vi "Agilent Channels.vi"(0 "file path (dialog if empty)":path=path "C:/NI-2010/Trunk/Dryer Wilt/Agilent Channel Assignment - Wilt.ini") -> (3 "Temperature Channels":T1[](array[typedef]), 4 "Station Data Headers":string[][](array[string]), 6 "Index Array":i32[][](array[numeric]), 8 "Agilent Channels Raw":T1[](array[typedef]), 10 "Agilent Channels To Read":T1[](array[typedef]), 14 "Start Buttons":T1[](array[typedef]), 15 "Agilent Channel Water Valves":T1[](array[typedef]))   [LabVIEW 2012]
uses:
  Agilent Channel Definition.ctl
  <vilib>/Utility/file.llb/Read From Spreadsheet File (string).vi
panel:
  out "Array":i32[](array[numeric])
  out "Agilent6 Channels":string[][](array[string])
  out "Agilent5 Channels":string[][](array[string])
  out "Agilent4 Channels":string[][](array[string])
  out "Agilent3 Channels":string[][](array[string])
  out "Agilent2 Channels":string[][](array[string])
  out "Agilent1 Channels":string[][](array[string])
  out "all rows":string[][](array[string])
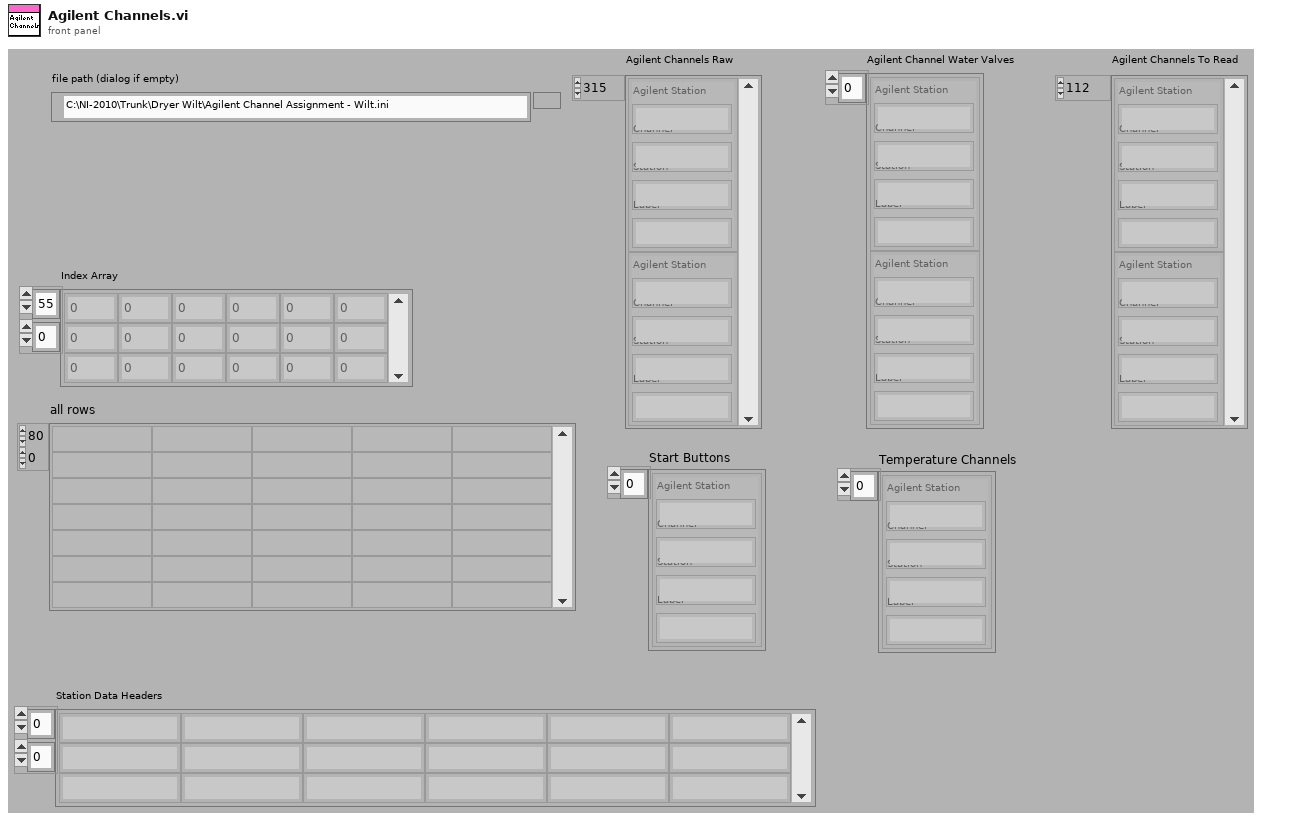
[diagram p1: front panel]
types:
  T1 = typedef "Agilent Channel Definition.ctl" = cluster{"Channel":string, "Station":string, "Label":string, "Agilent Station":string}
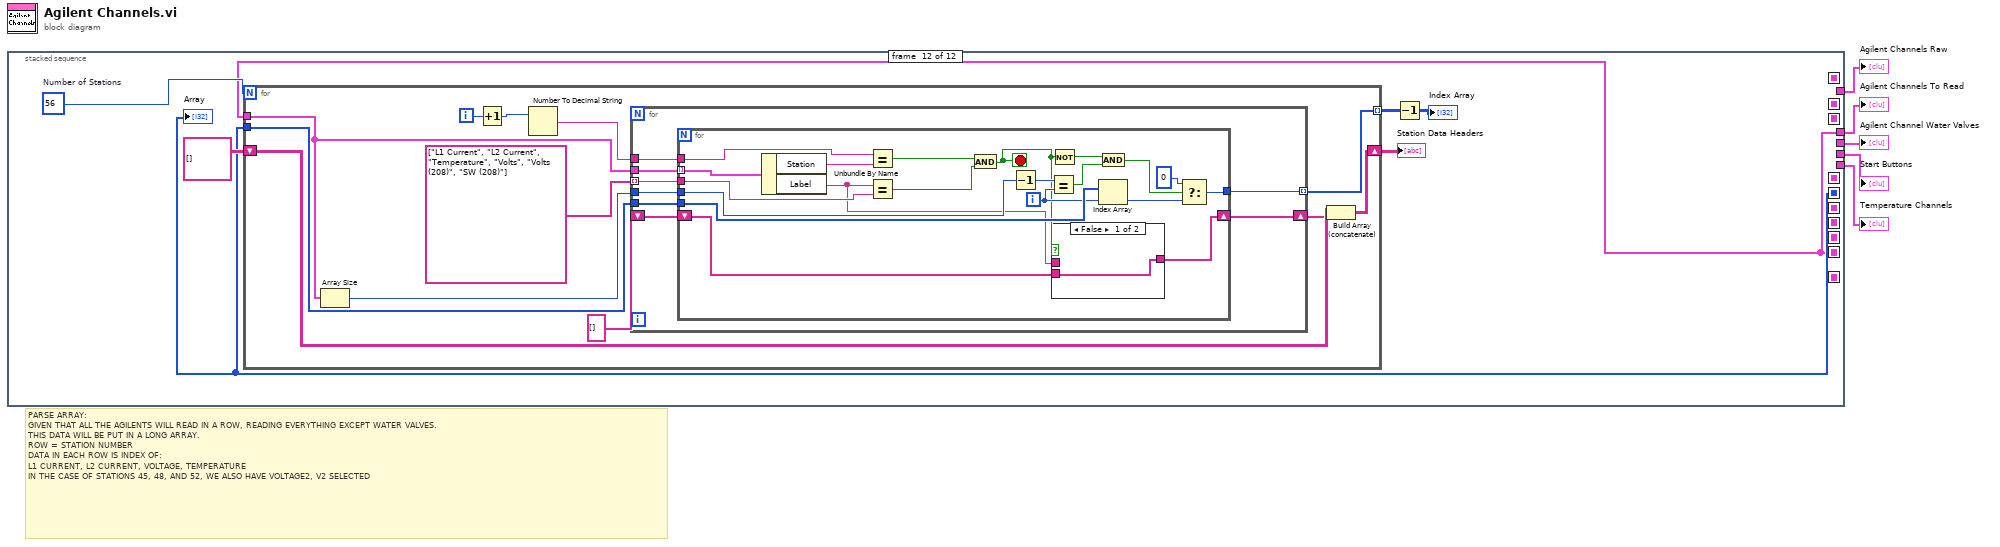
[diagram p0: block diagram]
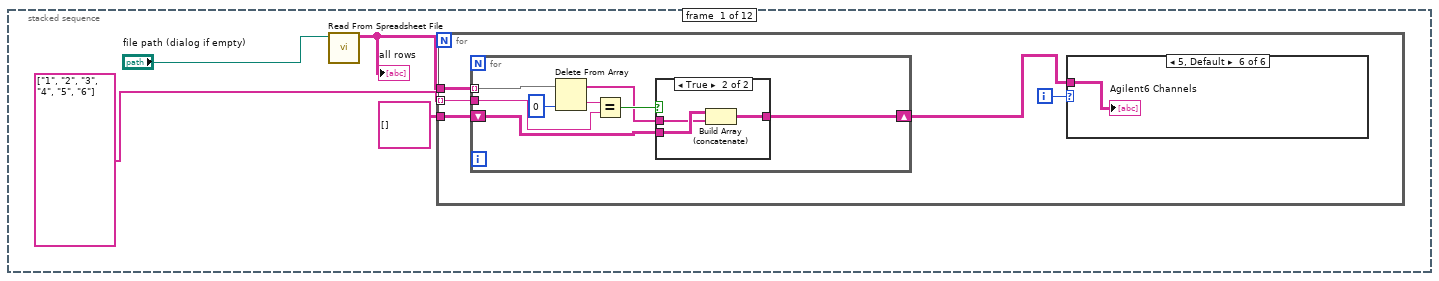
[diagram p2: hidden frame]
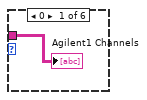
[diagram p3: hidden frame]
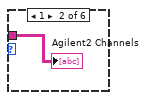
[diagram p4: hidden frame]
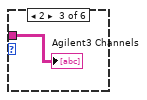
[diagram p5: hidden frame]
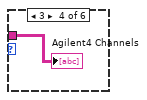
[diagram p6: hidden frame]
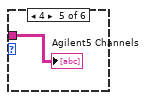
[diagram p7: hidden frame]
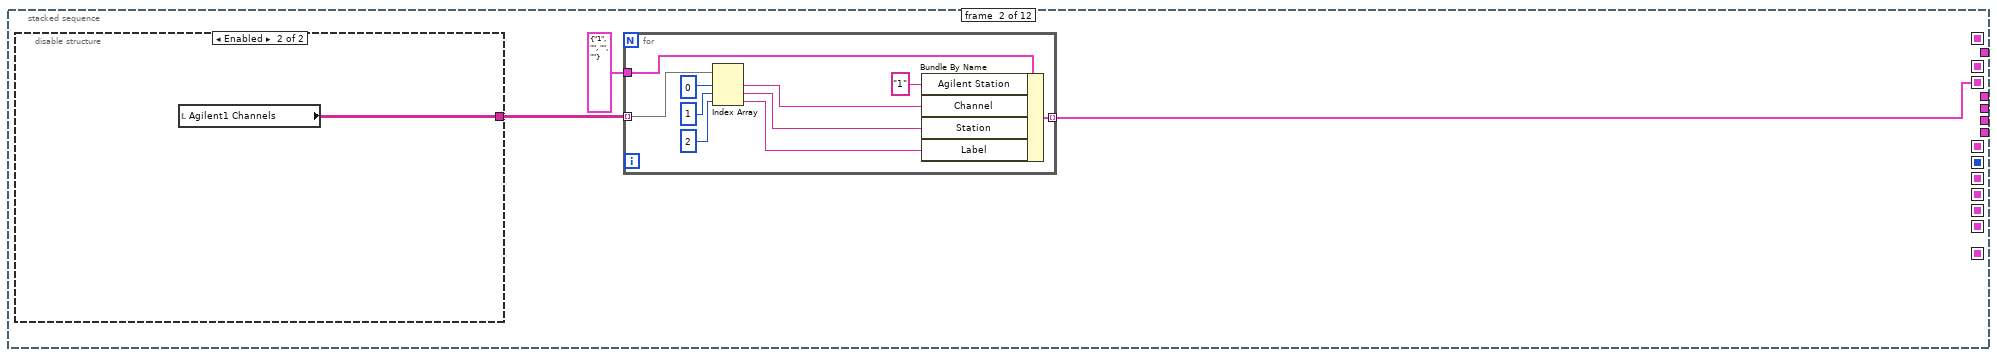
[diagram p9: hidden frame]
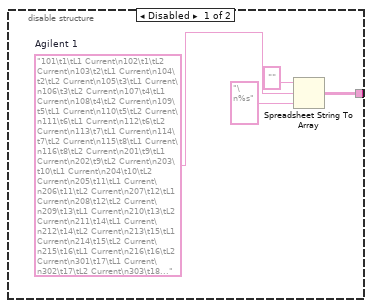
[diagram p10: hidden frame]
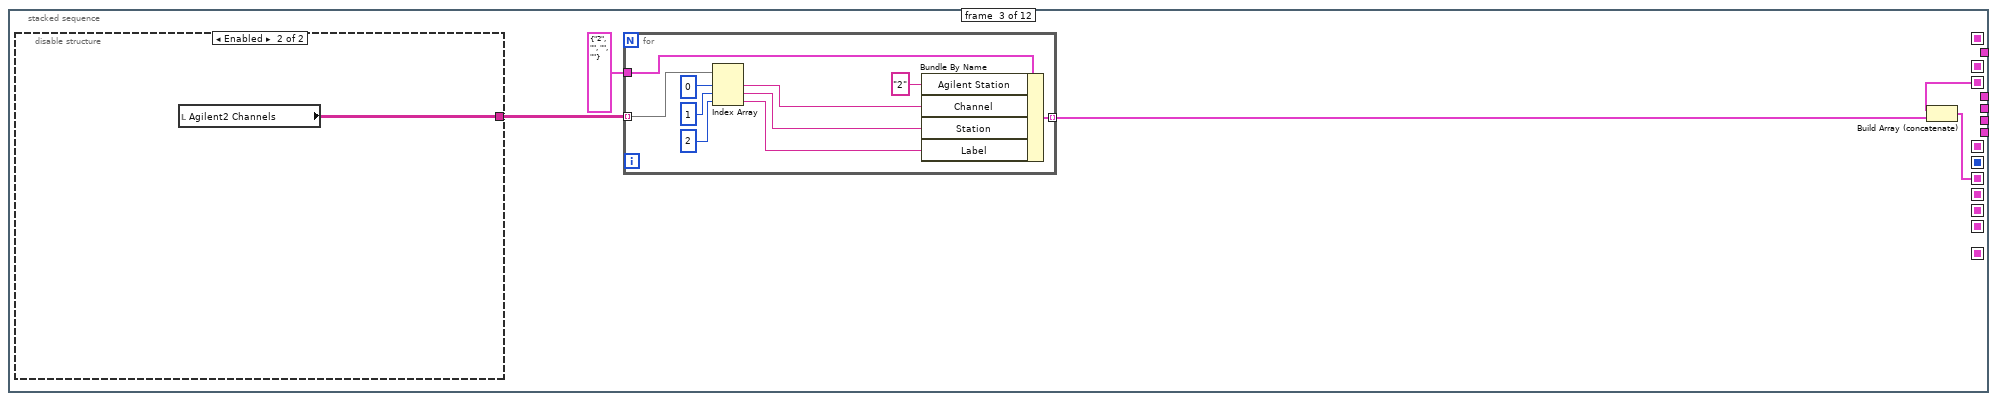
[diagram p11: hidden frame]
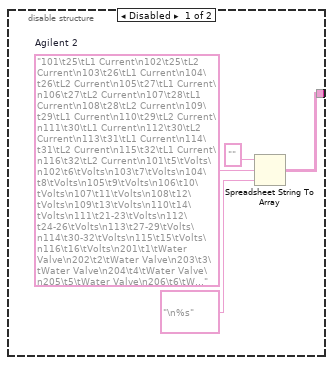
[diagram p12: hidden frame]
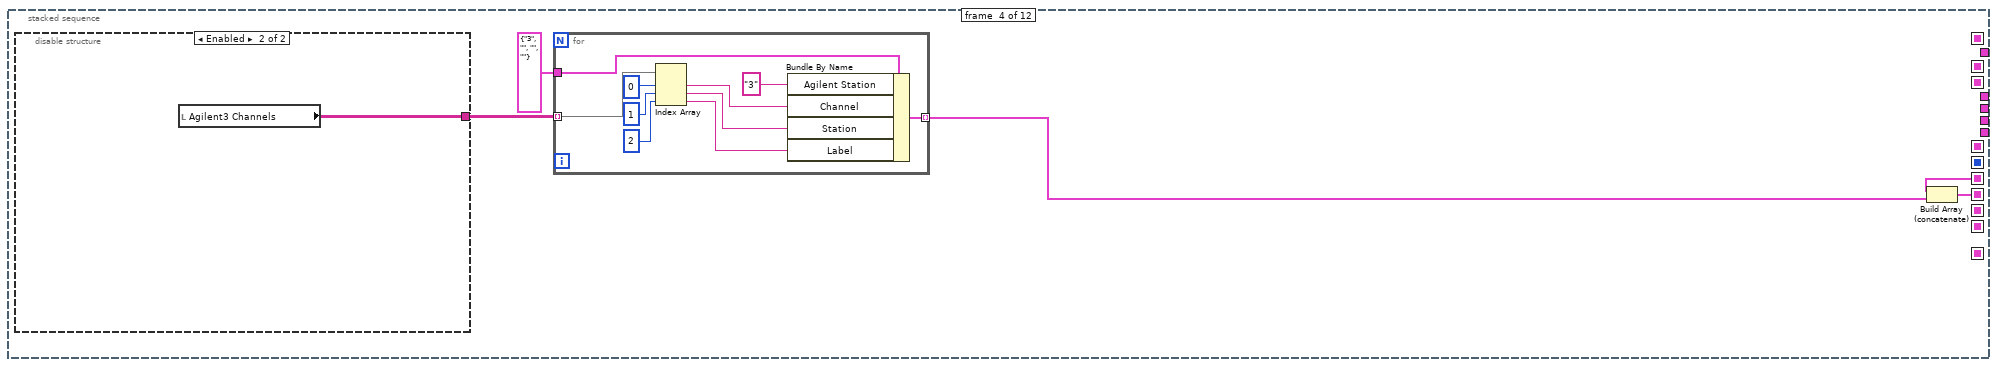
[diagram p13: hidden frame]
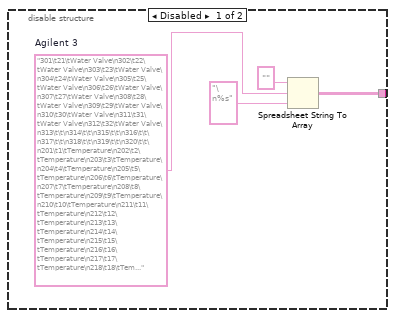
[diagram p14: hidden frame]
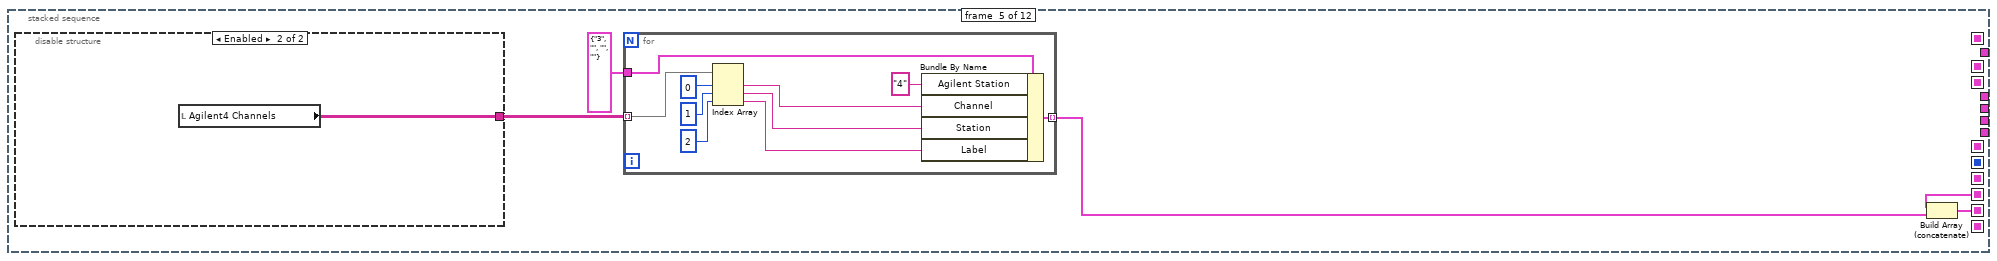
[diagram p15: hidden frame]
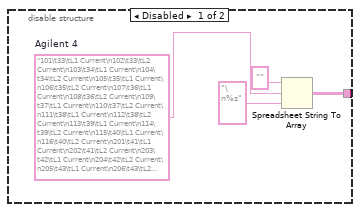
[diagram p16: hidden frame]
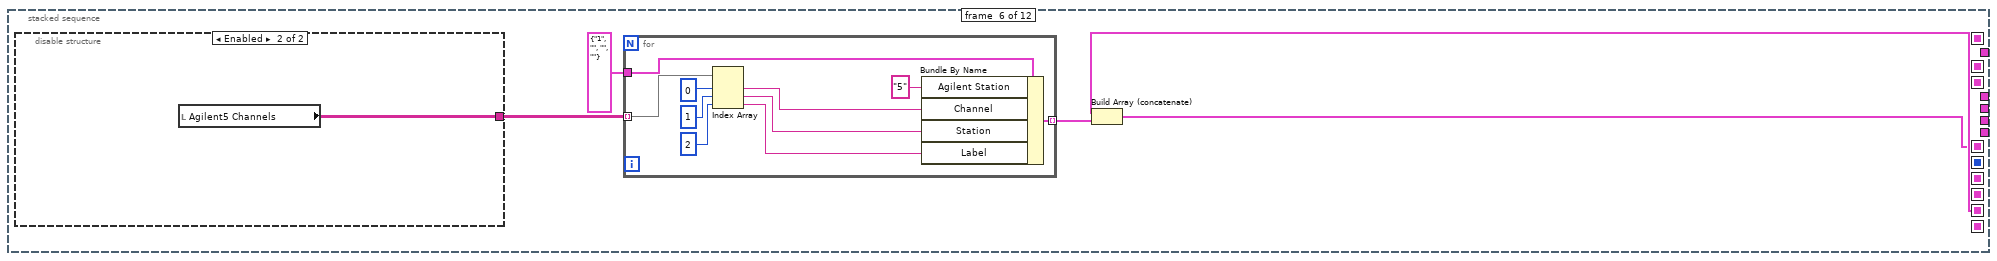
[diagram p17: hidden frame]
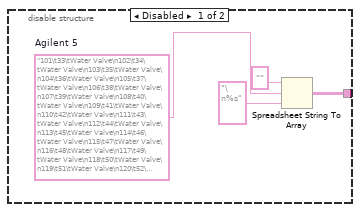
[diagram p18: hidden frame]
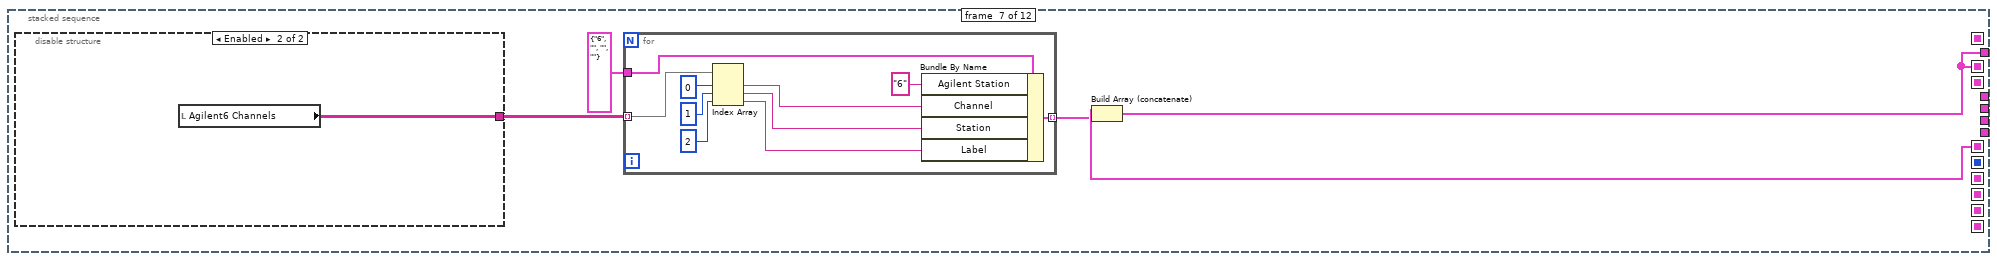
[diagram p19: hidden frame]
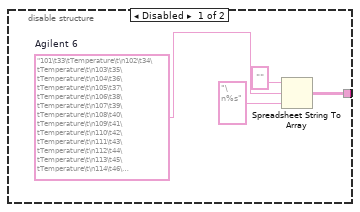
[diagram p20: hidden frame]
diagram:
  # "PARSE ARRAY:\nGIVEN THAT ALL THE AGILENTS WILL READ IN A ROW, READING EVERYTHING EXCEPT WATER VALVES.\nTHIS DATA WILL BE PUT IN A LONG ARRAY.\nROW = STATION NUMBER\nDATA IN EACH ROW IS INDEX OF:\nL1 CURRENT, L2 CURRENT, VOLTAGE, TEMPERATURE\nIN THE CASE OF STATIONS 45, 48, AND 52, WE ALSO HAVE VOLTAGE2, V2 SELECTED"
  n1 = stacked-sequence {
    seq-local: [_ w33 _ _ _ _ _ _ _ _ _ _] -> [_ _ w55 _ _ _ _ _ _ _ _ _]
    seq-local: [_ _ w54 _ _ _ _ _ _ _ _ _] -> [_ _ _ w75 _ _ _ _ _ _ _ _]
    seq-local: [_ _ _ w74 _ _ _ _ _ _ _ _] -> [_ _ _ _ w95 _ _ _ _ _ _ _]
    seq-local: [_ _ _ _ w94 _ _ _ _ _ _ _] -> [_ _ _ _ _ w115 _ _ _ _ _ _]
    seq-local: [_ _ _ _ _ w114 _ _ _ _ _ _] -> [_ _ _ _ _ _ w135 _ _ _ _ _]
    seq-local: [_ _ _ _ _ _ _ w154 _ _ _ _] -> [_ _ _ _ _ _ _ _ w173 _ _ _]
    seq-local: [_ _ _ _ _ _ _ _ _ _ w208 _] -> [_ _ _ _ _ _ _ _ _ _ _ w258]
    seq-local: [_ _ _ _ _ _ w131 _ _ _ _ _] -> [_ _ _ _ _ _ _ w153 _ w193 _ _]
    seq-local: [_ _ _ _ _ _ _ _ _ _ w206 _] -> [_ _ _ _ _ _ _ _ _ _ _ w261]
    seq-local: [_ _ _ _ _ _ _ _ w171 _ _ _] -> [_ _ _ _ _ _ _ _ _ _ w204 _]
    tunnel: [_ _ _ _ _ _ w131 _ _ _ _ _] -> w5
    tunnel: [_ _ _ _ _ _ _ _ _ _ _ w258] -> w4
    tunnel: [_ _ _ _ _ _ _ w151 _ _ _ _] -> w3
    tunnel: [_ _ _ _ _ _ _ _ w174 _ _ _] -> w2
    tunnel: [_ _ _ _ _ _ _ _ _ w191 _ _] -> w1
    frame #0 {
      n2 = call-poly <vilib>:"Read From Spreadsheet File.vi"("file path (dialog if empty)"="file path (dialog if empty)") -> ("all rows"=w8:string[][])  [unwired: 6 in, 4 out]
      "all rows" <- w8
      n3 = for {
        tunnel: w8 -> [w14]
        tunnel: string[][] [] -> [w12]
        tunnel: string[] ["1", "2", "3", "4", "5", "6"] -> [w11] mode=indexing
        i -> [w10]
        n4 = for {
          tunnel: w14 -> [w28] mode=indexing
          shift-right: [w24] -> w13
          shift-left: w12 -> [w23]
          tunnel: w11 -> [w21]
          n5 = Delete From Array(array=w28, index=0) -> (deleted portion=w26:string, array with subset deleted=w22:string[])  [unwired: 1 in]
          n6 = Equal?(x=w26, y=w21) -> (x = y?=w25:bool)
          n7 = case shown="True" w25 {
            tunnel: [w29 w32] -> w24
            tunnel: w23 -> [w29 w31]
            tunnel: w22 -> [_ w30]
            frame False {
            }
            frame True {
              n8 = Build Array (concatenate)(w31, w30) -> (w32:string[][])
            }
          }
        }
        n9 = case shown="5, Default" w10 {
          tunnel: w13 -> [w15 w16 w17 w18 w19 w20]
          frame 0 {
            "Agilent1 Channels" <- w15
          }
          frame 1 {
            "Agilent2 Channels" <- w16
          }
          frame 2 {
            "Agilent3 Channels" <- w17
          }
          frame 3 {
            "Agilent4 Channels" <- w18
          }
          frame 4 {
            "Agilent5 Channels" <- w19
          }
          frame 5, Default {
            "Agilent6 Channels" <- w20
          }
        }
      }
    }
    frame #1 {
      n10 = disable-structure shown="Enabled" {
        disable-tunnel: [w38 w40] -> w35
        frame Disabled {
          w36 = "101\t1\tL1 Current\n102\t1\tL2 Current\n103\t2\tL1 Current\n104\t2\tL2 Current\n105\t3\tL1 Current\n106\t3\tL2 Current\n107\t4\tL1 Current\n108\t4\tL2 Current\n109\t5\tL1 Current\n110\t5\tL2 Current\n111\t6\tL1 Current\n112\t6\tL2 Current\n113\t7\tL1 Current\n114\t7\tL2 Current\n115\t8\tL1 Current\n116\t8\tL2 Current\n201\t9\tL1 Current\n202\t9\tL2 Current\n203\t10\tL1 Current\n204\t10\tL2 Current\n205\t11\tL1 Current\n206\t11\tL2 Current\n207\t12\tL1 Current\n208\t12\tL2 Current\n209\t13\tL1 Current\n210\t13\tL2 Current\n211\t14\tL1 Current\n212\t14\tL2 Current\n213\t15\tL1 Current\n214\t15\tL2 Current\n215\t16\tL1 Current\n216\t16\tL2 Current\n301\t17\tL1 Current\n302\t17\tL2 Current\n303\t18\tL1 Current\n304\t18\tL2 Current\n305\t19\tL1 Current\n306\t19\tL2 Current\n307\t20\tL1 Current\n308\t20\tL2 Current\n309\t21\tL1 Current\n310\t21\tL2 Current\n311\t22\tL1 Current\n312\t22\tL2 Current\n313\t23\tL1 Current\n314\t23\tL2 Current\n315\t24\tL1 Current\n316\t24\tL2 Current"  # Agilent 1
          n11 = Spreadsheet String To Array(format string="", spreadsheet string=w36, array type (2D Dbl)="\n%s" ("format string")) -> (array=w38:string[][])  [unwired: 1 in]
        }
        frame Enabled {
          n12 = local read "Agilent1 Channels"() -> (w40:string[][])
        }
      }
      n13 = for {
        tunnel: w35 -> [w48] mode=indexing
        tunnel: T1 {"Channel"="1", "Station"="", "Label"="", "Agilent Station"=""} ("Agilent Channel Definition") -> [w50]
        tunnel: [w49] -> w33 mode=indexing
        n14 = Index Array(array=w48, index #1=0 ("index"), index #2=1 ("index"), index #3=2 ("index")) -> (element #1=w44:string, element #2=w43:string, element #3=w42:string)
        n15 = Bundle By Name(cluster=w50, "Agilent Station"="1" ("Channel"), "Channel"=w44, "Station"=w43, "Label"=w42) -> (w49:T1)
      }
    }
    frame #2 {
      n16 = disable-structure shown="Enabled" {
        disable-tunnel: [w56 w60] -> w51
        frame Disabled {
          w57 = "101\t25\tL1 Current\n102\t25\tL2 Current\n103\t26\tL1 Current\n104\t26\tL2 Current\n105\t27\tL1 Current\n106\t27\tL2 Current\n107\t28\tL1 Current\n108\t28\tL2 Current\n109\t29\tL1 Current\n110\t29\tL2 Current\n111\t30\tL1 Current\n112\t30\tL2 Current\n113\t31\tL1 Current\n114\t31\tL2 Current\n115\t32\tL1 Current\n116\t32\tL2 Current\n101\t5\tVolts\n102\t6\tVolts\n103\t7\tVolts\n104\t8\tVolts\n105\t9\tVolts\n106\t10\tVolts\n107\t11\tVolts\n108\t12\tVolts\n109\t13\tVolts\n110\t14\tVolts\n111\t21-23\tVolts\n112\t24-26\tVolts\n113\t27-29\tVolts\n114\t30-32\tVolts\n115\t15\tVolts\n116\t16\tVolts\n201\t1\tWater Valve\n202\t2\tWater Valve\n203\t3\tWater Valve\n204\t4\tWater Valve\n205\t5\tWater Valve\n206\t6\tWater Valve\n207\t7\tWater Valve\n208\t8\tWater Valve\n209\t9\tWater Valve\n210\t10\tWater Valve\n211\t11\tWater Valve\n212\t12\tWater Valve\n213\t13\tWater Valve\n214\t14\tWater Valve\n215\t15\tWater Valve\n216\t16\tWater Valve\n217\t17\tWater Valve\n218\t18\tWater Valve\n219\t19\tWater Valve\n220\t20\tWater Valve"  # Agilent 2
          n17 = Spreadsheet String To Array(format string="", spreadsheet string=w57, array type (2D Dbl)="\n%s" ("format string")) -> (array=w56:string[][])  [unwired: 1 in]
        }
        frame Enabled {
          n18 = local read "Agilent2 Channels"() -> (w60:string[][])
        }
      }
      n19 = for {
        tunnel: w51 -> [w68] mode=indexing
        tunnel: T1 {"Channel"="2", "Station"="", "Label"="", "Agilent Station"=""} ("Agilent Channel Definition") -> [w70]
        tunnel: [w69] -> w53 mode=indexing
        n20 = Index Array(array=w68, index #1=0 ("index"), index #2=1 ("index"), index #3=2 ("index")) -> (element #1=w64:string, element #2=w63:string, element #3=w62:string)
        n21 = Bundle By Name(cluster=w70, "Agilent Station"="2" ("Channel"), "Channel"=w64, "Station"=w63, "Label"=w62) -> (w69:T1)
      }
      n22 = Build Array (concatenate)(w55, w53) -> (w54:T1[])
    }
    frame #3 {
      n23 = disable-structure shown="Enabled" {
        disable-tunnel: [w76 w80] -> w71
        frame Disabled {
          w77 = "301\t21\tWater Valve\n302\t22\tWater Valve\n303\t23\tWater Valve\n304\t24\tWater Valve\n305\t25\tWater Valve\n306\t26\tWater Valve\n307\t27\tWater Valve\n308\t28\tWater Valve\n309\t29\tWater Valve\n310\t30\tWater Valve\n311\t31\tWater Valve\n312\t32\tWater Valve\n313\t\t\n314\t\t\n315\t\t\n316\t\t\n317\t\t\n318\t\t\n319\t\t\n320\t\t\n201\t1\tTemperature\n202\t2\tTemperature\n203\t3\tTemperature\n204\t4\tTemperature\n205\t5\tTemperature\n206\t6\tTemperature\n207\t7\tTemperature\n208\t8\tTemperature\n209\t9\tTemperature\n210\t10\tTemperature\n211\t11\tTemperature\n212\t12\tTemperature\n213\t13\tTemperature\n214\t14\tTemperature\n215\t15\tTemperature\n216\t16\tTemperature\n217\t17\tTemperature\n218\t18\tTemperature\n219\t19\tTemperature\n220\t20\tTemperature\n301\t21\tTemperature\n302\t22\tTemperature\n303\t23\tTemperature\n304\t24\tTemperature\n305\t25\tTemperature\n306\t26\tTemperature\n307\t27\tTemperature\n308\t28\tTemperature\n309\t29\tTemperature\n310\t30\tTemperature\n311\t31\tTemperature\n312\t32\tTemperature\n313\t1\tVolts\n314\t2\tVolts\n315\t3\tVolts\n316\t4\tVolts"  # Agilent 3
          n24 = Spreadsheet String To Array(format string="", spreadsheet string=w77, array type (2D Dbl)="\n%s" ("format string")) -> (array=w76:string[][])  [unwired: 1 in]
        }
        frame Enabled {
          n25 = local read "Agilent3 Channels"() -> (w80:string[][])
        }
      }
      n26 = for {
        tunnel: w71 -> [w88] mode=indexing
        tunnel: T1 {"Channel"="3", "Station"="", "Label"="", "Agilent Station"=""} ("Agilent Channel Definition") -> [w90]
        tunnel: [w89] -> w73 mode=indexing
        n27 = Index Array(array=w88, index #1=0 ("index"), index #2=1 ("index"), index #3=2 ("index")) -> (element #1=w84:string, element #2=w83:string, element #3=w82:string)
        n28 = Bundle By Name(cluster=w90, "Agilent Station"="3" ("Channel"), "Channel"=w84, "Station"=w83, "Label"=w82) -> (w89:T1)
      }
      n29 = Build Array (concatenate)(w75, w73) -> (w74:T1[])
    }
    frame #4 {
      n30 = disable-structure shown="Enabled" {
        disable-tunnel: [w96 w100] -> w93
        frame Disabled {
          w97 = "101\t33\tL1 Current\n102\t33\tL2 Current\n103\t34\tL1 Current\n104\t34\tL2 Current\n105\t35\tL1 Current\n106\t35\tL2 Current\n107\t36\tL1 Current\n108\t36\tL2 Current\n109\t37\tL1 Current\n110\t37\tL2 Current\n111\t38\tL1 Current\n112\t38\tL2 Current\n113\t39\tL1 Current\n114\t39\tL2 Current\n115\t40\tL1 Current\n116\t40\tL2 Current\n201\t41\tL1 Current\n202\t41\tL2 Current\n203\t42\tL1 Current\n204\t42\tL2 Current\n205\t43\tL1 Current\n206\t43\tL2 Current\n207\t44\tL1 Current\n208\t44\tL2 Current\n209\t45\tL1 Current\n210\t45\tL2 Current\n211\t46\tL1 Current\n212\t46\tL2 Current\n213\t47\tL1 Current\n214\t47\tL2 Current\n215\t48\tL1 Current\n216\t48\tL2 Current\n301\t49\tL1 Current\n302\t49\tL2 Current\n303\t50\tL1 Current\n304\t50\tL2 Current\n305\t51\tL1 Current\n306\t51\tL2 Current\n307\t52\tL1 Current\n308\t52\tL2 Current\n309\t53\tL1 Current\n310\t53\tL2 Current\n311\t54\tL1 Current\n312\t54\tL2 Current\n313\t55\tL1 Current\n314\t55\tL2 Current\n315\t56\tL1 Current\n316\t56\tL2 Current"  # Agilent 4
          n31 = Spreadsheet String To Array(format string="", spreadsheet string=w97, array type (2D Dbl)="\n%s" ("format string")) -> (array=w96:string[][])  [unwired: 1 in]
        }
        frame Enabled {
          n32 = local read "Agilent4 Channels"() -> (w100:string[][])
        }
      }
      n33 = for {
        tunnel: w93 -> [w108] mode=indexing
        tunnel: T1 {"Channel"="3", "Station"="", "Label"="", "Agilent Station"=""} ("Agilent Channel Definition") -> [w110]
        tunnel: [w109] -> w92 mode=indexing
        n34 = Index Array(array=w108, index #1=0 ("index"), index #2=1 ("index"), index #3=2 ("index")) -> (element #1=w104:string, element #2=w103:string, element #3=w102:string)
        n35 = Bundle By Name(cluster=w110, "Agilent Station"="4" ("Channel"), "Channel"=w104, "Station"=w103, "Label"=w102) -> (w109:T1)
      }
      n36 = Build Array (concatenate)(w95, w92) -> (w94:T1[])
    }
    frame #5 {
      n37 = disable-structure shown="Enabled" {
        disable-tunnel: [w117 w120] -> w113
        frame Disabled {
          w116 = "101\t33\tWater Valve\n102\t34\tWater Valve\n103\t35\tWater Valve\n104\t36\tWater Valve\n105\t37\tWater Valve\n106\t38\tWater Valve\n107\t39\tWater Valve\n108\t40\tWater Valve\n109\t41\tWater Valve\n110\t42\tWater Valve\n111\t43\tWater Valve\n112\t44\tWater Valve\n113\t45\tWater Valve\n114\t46\tWater Valve\n115\t47\tWater Valve\n116\t48\tWater Valve\n117\t49\tWater Valve\n118\t50\tWater Valve\n119\t51\tWater Valve\n120\t52\tWater Valve\n201\t53\tWater Valve\n202\t54\tWater Valve\n203\t55\tWater Valve\n204\t56\tWater Valve"  # Agilent 5
          n38 = Spreadsheet String To Array(format string="", spreadsheet string=w116, array type (2D Dbl)="\n%s" ("format string")) -> (array=w117:string[][])  [unwired: 1 in]
        }
        frame Enabled {
          n39 = local read "Agilent5 Channels"() -> (w120:string[][])
        }
      }
      n40 = for {
        tunnel: w113 -> [w128] mode=indexing
        tunnel: T1 {"Channel"="1", "Station"="", "Label"="", "Agilent Station"=""} ("Agilent Channel Definition") -> [w130]
        tunnel: [w129] -> w111 mode=indexing
        n41 = Index Array(array=w128, index #1=0 ("index"), index #2=1 ("index"), index #3=2 ("index")) -> (element #1=w124:string, element #2=w123:string, element #3=w122:string)
        n42 = Bundle By Name(cluster=w130, "Agilent Station"="5" ("Channel"), "Channel"=w124, "Station"=w123, "Label"=w122) -> (w129:T1)
      }
      n43 = Build Array (concatenate)(w115, w111) -> (w114:T1[])
    }
    frame #6 {
      n44 = disable-structure shown="Enabled" {
        disable-tunnel: [w137 w140] -> w134
        frame Disabled {
          w136 = "101\t33\tTemperature\t\n102\t34\tTemperature\t\n103\t35\tTemperature\t\n104\t36\tTemperature\t\n105\t37\tTemperature\t\n106\t38\tTemperature\t\n107\t39\tTemperature\t\n108\t40\tTemperature\t\n109\t41\tTemperature\t\n110\t42\tTemperature\t\n111\t43\tTemperature\t\n112\t44\tTemperature\t\n113\t45\tTemperature\t\n114\t46\tTemperature\t\n115\t47\tTemperature\t\n116\t48\tTemperature\t\n117\t49\tTemperature\t\n118\t50\tTemperature\t\n119\t51\tTemperature\t\n120\t52\tTemperature\t\n201\t53\tTemperature\t\n202\t54\tTemperature\t\n203\t55\tTemperature\t\n204\t56\tTemperature\t\n205\t33-35\tVolts\t\n206\t36-38\tVolts\t\n207\t39-40\tVolts\t\n208\t42-44\tVolts\t\n209\t45-47\tVolts\t\n210\t45\tVolts (208)\t\n211\t45\tSW (208)\t\n212\t48-50\tVolts\t\n213\t48\tSW (208)\t\n214\t51\tVolts\t\n215\t51\tSW (208)\t\n216\t54-56\tVolts\t"  # Agilent 6
          n45 = Spreadsheet String To Array(format string="", spreadsheet string=w136, array type (2D Dbl)="\n%s" ("format string")) -> (array=w137:string[][])  [unwired: 1 in]
        }
        frame Enabled {
          n46 = local read "Agilent6 Channels"() -> (w140:string[][])
        }
      }
      n47 = for {
        tunnel: w134 -> [w148] mode=indexing
        tunnel: T1 {"Channel"="6", "Station"="", "Label"="", "Agilent Station"=""} ("Agilent Channel Definition") -> [w150]
        tunnel: [w149] -> w132 mode=indexing
        n48 = Index Array(array=w148, index #1=0 ("index"), index #2=1 ("index"), index #3=2 ("index")) -> (element #1=w144:string, element #2=w143:string, element #3=w142:string)
        n49 = Bundle By Name(cluster=w150, "Agilent Station"="6" ("Channel"), "Channel"=w144, "Station"=w143, "Label"=w142) -> (w149:T1)
      }
      n50 = Build Array (concatenate)(w135, w132) -> (w131:T1[])
    }
    frame #7 {
      w152 = T1[] []
      # "Build Array without water valve entries"
      # "PARSE ARRAY:\nGIVEN THAT ALL THE AGILENTS WILL READ IN A ROW, READING EVERYTHING EXCEPT WATER VALVES.\nTHIS DATA WILL BE PUT IN A LONG ARRAY.\nROW = STATION NUMBER\nDATA IN EACH ROW IS INDEX OF:\nL1 CURRENT, L2 CURRENT, VOLTAGE, TEMPERATURE\nIN THE CASE OF STATIONS 45, 48, AND 52, WE ALSO HAVE VOLTAGE2, V2 SELECTED"
      n51 = for {
        tunnel: w153 -> [w158] mode=indexing
        shift-right: [w159] -> w154
        shift-left: w152 -> [w156]
        shift-right: [w155] -> w151
        shift-left: w152 -> [w157]
        n52 = Unbundle By Name(w158) -> ("Label"=w162:string)
        n53 = Equal?(x=w162, y="Water Valve") -> (x = y?=w160:bool)
        n54 = case shown="False" w160 {
          tunnel: w158 -> [w166 w167]
          tunnel: [w165 w170] -> w159
          tunnel: w156 -> [w164 w170]
          tunnel: w157 -> [w163 w169]
          tunnel: [w163 w168] -> w155
          frame False {
            n55 = Build Array (concatenate)(w164, w166) -> (w165:T1[])
          }
          frame True {
            n56 = Build Array (concatenate)(w169, w167) -> (w168:T1[])
          }
        }
      }
    }
    frame #8 {
      w172 = T1[] []
      # "Build Array with start button entries"
      # "PARSE ARRAY:\nGIVEN THAT ALL THE AGILENTS WILL READ IN A ROW, READING EVERYTHING EXCEPT WATER VALVES.\nTHIS DATA WILL BE PUT IN A LONG ARRAY.\nROW = STATION NUMBER\nDATA IN EACH ROW IS INDEX OF:\nL1 CURRENT, L2 CURRENT, VOLTAGE, TEMPERATURE\nIN THE CASE OF STATIONS 45, 48, AND 52, WE ALSO HAVE VOLTAGE2, V2 SELECTED"
      n57 = for {
        tunnel: w173 -> [w179] mode=indexing
        shift-right: [w177] -> w174
        shift-left: w172 -> [w178]
        shift-right: [w175] -> w171
        shift-left: w172 -> [w176]
        n58 = Unbundle By Name(w179) -> ("Label"=w182:string)
        n59 = Equal?(x=w182, y="Start Button") -> (x = y?=w180:bool)
        n60 = case shown="False" w180 {
          tunnel: w179 -> [w184 w188]
          tunnel: w178 -> [w186 w190]
          tunnel: [w186 w189] -> w177
          tunnel: w176 -> [w185 w187]
          tunnel: [w183 w187] -> w175
          frame False {
            n61 = Build Array (concatenate)(w185, w184) -> (w183:T1[])
          }
          frame True {
            n62 = Build Array (concatenate)(w190, w188) -> (w189:T1[])
          }
        }
      }
    }
    frame #9 {
      # "Build Array with Temperature entries"
      # "PARSE ARRAY:\nGIVEN THAT ALL THE AGILENTS WILL READ IN A ROW, READING EVERYTHING EXCEPT WATER VALVES.\nTHIS DATA WILL BE PUT IN A LONG ARRAY.\nROW = STATION NUMBER\nDATA IN EACH ROW IS INDEX OF:\nL1 CURRENT, L2 CURRENT, VOLTAGE, TEMPERATURE\nIN THE CASE OF STATIONS 45, 48, AND 52, WE ALSO HAVE VOLTAGE2, V2 SELECTED"
      n63 = for {
        tunnel: w193 -> [w196] mode=indexing
        shift-right: [w194] -> w191
        shift-left: T1[] [] -> [w195]
        n64 = Unbundle By Name(w196) -> ("Label"=w199:string)
        n65 = Equal?(x=w199, y="Temperature") -> (x = y?=w197:bool)
        n66 = case shown="True" w197 {
          tunnel: w196 -> [_ w201]
          tunnel: w195 -> [w200 w203]
          tunnel: [w200 w202] -> w194
          frame False {
          }
          frame True {
            n67 = Build Array (concatenate)(w203, w201) -> (w202:T1[])
          }
        }
      }
    }
    frame #10 {
      # "Clean up Station Entries.  If station has - in it, i.e. 33-35, clean it up to 3 entries, 33,34, and 35.\nSkip Blanks"
      n68 = for {
        tunnel: w204 -> [w216] mode=indexing
        shift-right: [w215] -> w208
        shift-left: T1[] [] -> [w214]
        shift-right: [w213] -> w206
        shift-left: i32[] [] -> [w212]
        shift-right: [w210] -> _
        shift-left: 0 -> [w211]
        n69 = Unbundle By Name(w216) -> ("Station"=w221:string)
        n70 = Match Pattern(string=w221, regular expression="-") -> (before substring=w217:string, offset past match=w219:i32)  [unwired: 1 in, 2 out]
        n71 = Greater Or Equal To 0?(x=w219) -> (x >= 0?=w218:bool)
        n72 = case shown="True" w218 {
          tunnel: w217 -> [w228 w254]
          tunnel: w216 -> [w231 w249]
          tunnel: [w229 w252] -> w215
          tunnel: w214 -> [w230 w251]
          tunnel: w211 -> [w225 w243]
          tunnel: [w224 w244] -> w213
          tunnel: w212 -> [w223 w245]
          tunnel: [w222 w242] -> w210
          frame False {
            n73 = Equal?(x=w228, y="") -> (x = y?=w226:bool)
            n74 = case shown="False" w226 {
              tunnel: w231 -> [w238 _]
              tunnel: w230 -> [w237 w241]
              tunnel: [w236 w241] -> w229
              tunnel: w225 -> [w233 w239]
              tunnel: [w235 w240] -> w224
              tunnel: w223 -> [w234 w240]
              tunnel: [w232 w239] -> w222
              frame False {
                n75 = Increment(x=w233) -> (x+1=w232:i32)
                n76 = Build Array (concatenate)(w237, w238) -> (w236:T1[])
                n77 = Build Array (concatenate)(w234, w232) -> (w235:i32[])
              }
              frame True {
              }
            }
          }
          frame True {
            n78 = Bundle By Name(cluster=w249, "Station"=w254) -> (w253:T1)
            n79 = Decimal String To Number(string=w254) -> (number=w257:i32)  [unwired: 2 in, 1 out]
            n80 = Increment(x=w243) -> (x+1=w242:i32)
            n81 = Build Array (concatenate)(w245, w242, w242, w242) -> (w244:i32[])
            n82 = Increment(x=w257) -> (x+1=w256:i32)
            n83 = Increment(x=w256) -> (x+1=w255:i32)
            n84 = Number To Decimal String(number=w256) -> (decimal integer string=w248:string)  [unwired: 1 in]
            n85 = Number To Decimal String(number=w255) -> (decimal integer string=w250:string)  [unwired: 1 in]
            n86 = Bundle By Name(cluster=w249, "Station"=w248) -> (w246:T1)
            n87 = Bundle By Name(cluster=w249, "Station"=w250) -> (w247:T1)
            n88 = Build Array (concatenate)(w251, w253, w246, w247) -> (w252:T1[])
          }
        }
      }
    }
    frame #11 {
      w264 = 56  # Number of Stations
      n89 = for {
        N: w264 -> [_]
        tunnel: w258 -> [w268]
        tunnel: [w273] -> w259 mode=indexing
        shift-right: [w271] -> w262
        shift-left: string[][] [] -> [w270]
        tunnel: w261 -> [w269]
        i -> [w276]
        n90 = Array Size(array=w268) -> (size(s)=w267:i32)
        n91 = Increment(x=w276) -> (x+1=w275:i32)
        n92 = Number To Decimal String(number=w275) -> (decimal integer string=w274:string)  [unwired: 1 in]
        n93 = for {
          tunnel: w268 -> [w284]
          tunnel: string[] ["L1 Current", "L2 Current", "Temperature", "Volts", "Volts (208)", "SW (208)"] -> [w282] mode=indexing
          tunnel: w274 -> [w283]
          tunnel: [w281] -> w273 mode=indexing
          tunnel: w269 -> [w280]
          tunnel: w267 -> [w279]
          shift-right: [w277] -> w265
          shift-left: string[] [] -> [w278]
          n94 = for {
            tunnel: w284 -> [w304] mode=indexing
            tunnel: w283 -> [w286]
            tunnel: w282 -> [w302]
            tunnel: [w298] -> w281
            tunnel: w280 -> [w300]
            tunnel: w279 -> [w299]
            shift-right: [w289] -> w277
            shift-left: w278 -> [w290]
            i -> [w291]
            stop <- w287 stop-if-true
            n95 = Unbundle By Name(w304) -> ("Station"=w285:string, "Label"=w288:string)
            n96 = Equal?(x=w286, y=w285) -> (x = y?=w303:bool)
            n97 = Equal?(x=w288, y=w302) -> (x = y?=w301:bool)
            n98 = And(x=w303, y=w301) -> (x .and. y?=w287:bool)
            n99 = Decrement(x=w299) -> (x-1=w292:i32)
            n100 = Equal?(x=w292, y=w291) -> (x = y?=w295:bool)
            n101 = Not(x=w287) -> (.not. x?=w293:bool)
            n102 = case shown="False" w287 {
              tunnel: w290 -> [w305 w308]
              tunnel: [w305 w307] -> w289
              tunnel: w288 -> [_ w306]
              frame False {
              }
              frame True {
                n103 = Build Array (concatenate)(w308, w306) -> (w307:string[])
              }
            }
            n104 = Index Array(array=w300, index=w291) -> (element=w297:i32)
            n105 = And(x=w293, y=w295) -> (x .and. y?=w294:bool)
            n106 = Select(t=0, s=w294, f=w297) -> (s? t:f=w298:i32)
          }
        }
        n107 = Build Array (concatenate)(w270, w265) -> (w271:string[][])
      }
      "Station Data Headers" <- w262
      n108 = Decrement(x=w259) -> (x-1=→"Index Array":i32[][])
      "Array" <- w261
    }
  }
  "Agilent Channels Raw" <- w5
  "Agilent Channels To Read" <- w4
  "Agilent Channel Water Valves" <- w3
  "Start Buttons" <- w2
  "Temperature Channels" <- w1
